vi "AudioStreamer.IsOutputDeviceValid.vi"(1 "device":string) -> (0 "result":string)   [LabVIEW 2020]
uses:
  <vilib>/Dataflow_G/G-Audio/G-Audio.lvlib
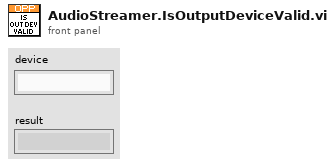
[diagram p1: front panel]
types:
  T1 = typedef "G-Audio.lvlib/Audio Device Info.ctl" = cluster{"Name":string, "ID":u8[], "Device Type":T2, "Default":bool, "Native Data Formats":T3[]}
  T2 = typedef "G-Audio.lvlib/Audio Device Type.ctl" = enum16{"(None)", "Playback", "Capture", "Duplex", "Loopback"}
  T3 = typedef "G-Audio.lvlib/Audio Device Native Data Format.ctl" = cluster{"Format":T4, "Channels":u32, "Sample Rate (Hz)":u32, "Exclusive Mode":bool}
  T4 = typedef "G-Audio.lvlib/Audio Device Format.ctl" = enum16{"Native", "U8", "I16", "I32", "SGL"}
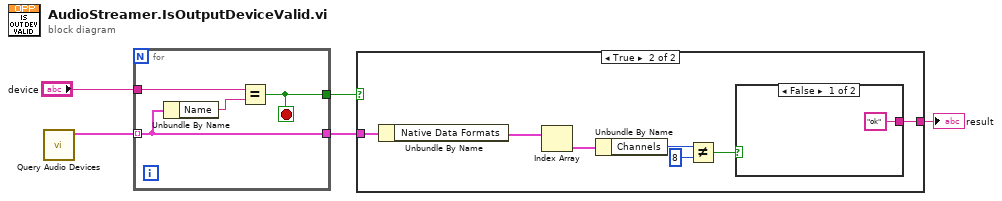
[diagram p0: block diagram]
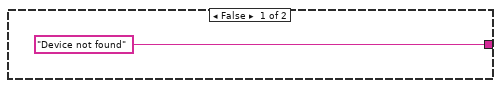
[diagram p2: hidden frame]
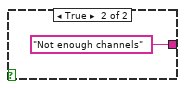
[diagram p3: hidden frame]
diagram:
  n1 = call <vilib>:"Query Audio Devices.vi"() -> ("Playback Devices"=w5:T1[])  [unwired: 7 in, 4 out]
  n2 = for {
    tunnel: w5 -> [w6] mode=indexing
    tunnel: "device" -> [w8]
    tunnel: [w7] -> w2
    tunnel: [w6] -> w3
    stop <- w7 stop-if-true
    n3 = Unbundle By Name(w6) -> ("Name"=w9:string)
    n4 = Equal?(x=w8, y=w9) -> (x = y?=w7:bool)
  }
  n5 = case shown="True" w2 {
    tunnel: w3 -> [_ w17]
    tunnel: ["Device not found" w11] -> w1
    frame False {
    }
    frame True {
      n6 = Unbundle By Name(w17) -> ("Native Data Formats"=w16:T3[])
      n7 = Index Array(array=w16) -> (element=w15:T3)  [unwired: 1 in]
      n8 = Unbundle By Name(w15) -> ("Channels"=w14:u32)
      n9 = Not Equal?(x=w14, y=u32 8) -> (x != y?=w12:bool)
      n10 = case shown="False" w12 {
        tunnel: ["ok" "Not enough channels"] -> w11
        frame False {
        }
        frame True {
        }
      }
    }
  }
  "result" <- w1
